vi "Log.vi"(7 "Message":string, 8 "error in (no error)":errorcluster, 10 "Level":T1, 11 "Logger in":refnum<class "Logger.lvclass">) -> (0 "error out":errorcluster, 3 "Logger out":refnum<class "Logger.lvclass">)   [LabVIEW 2022 SP3, in "Logger.lvlib" / "Logger.lvclass"]
uses:
  Logger.lvclass
  Logger.lvclass/Logger.ctl
  _Level.ctl
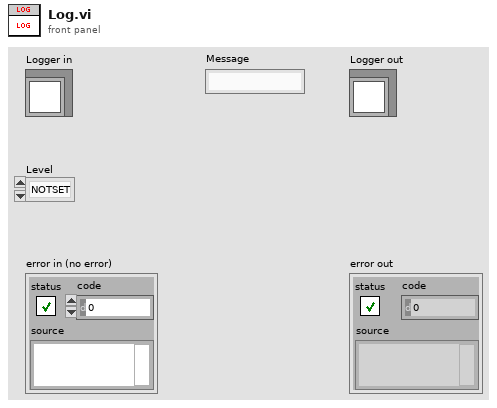
[diagram p1: front panel]
types:
  T1 = typedef "Logger.lvlib/Logger.lvclass/_Level.ctl" = enum16{"NOTSET", "DEBUG", "INFO", "WARNING", "ERROR", "CRITICAL"}
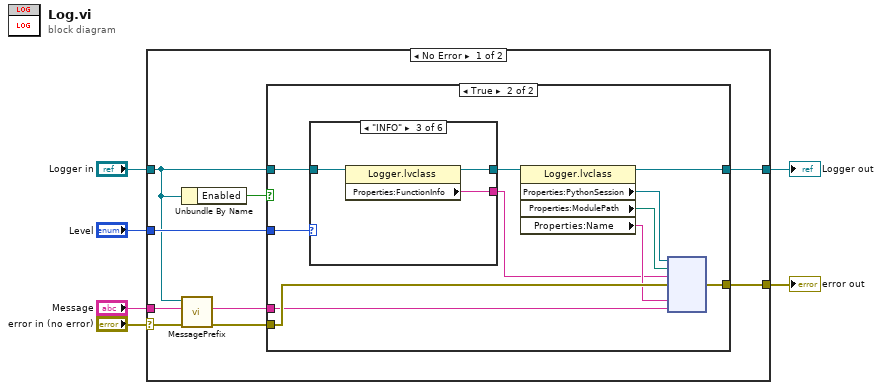
[diagram p0: block diagram]
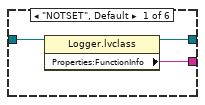
[diagram p3: hidden frame]
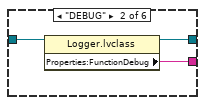
[diagram p4: hidden frame]
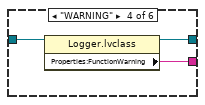
[diagram p5: hidden frame]
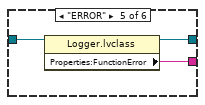
[diagram p6: hidden frame]
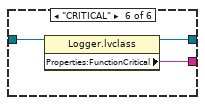
[diagram p7: hidden frame]
diagram:
  n1 = case shown="No Error" "error in (no error)" {
    selector: "error in (no error)" -> [w11 w48]
    tunnel: [w14 w48] -> w2
    tunnel: [w15 w47] -> w4
    tunnel: "Logger in" -> [w10 w47]
    tunnel: "Message" -> [w8 _]
    tunnel: "Level" -> [w12 _]
    frame No Error {
      n2 = Unbundle By Name(w10) -> ("Enabled"=w13:bool)
      n3 = call-dynamic "MessagePrefix.vi"("error in (no error)"=w11, "Message in"=w8, "Logger in"=w10) -> ("error out"=w7:errorcluster, "Message out"=w9:string)  [unwired: 6 in, 1 out]
      n4 = case shown="True" w13 {
        tunnel: [w17 w28] -> w15
        tunnel: w7 -> [w16 w27]
        tunnel: [w16 w26] -> w14
        tunnel: w9 -> [_ w23]
        tunnel: w10 -> [w17 w19]
        tunnel: w12 -> [_ w21]
        frame False {
        }
        frame True {
          n5 = case shown="\"INFO\"" w21 {
            tunnel: [w30 w33 w36 w39 w42 w45] -> w20
            tunnel: w19 -> [w31 w34 w37 w40 w43 w46]
            tunnel: [w29 w32 w35 w38 w41 w44] -> w18
            frame "NOTSET", Default {
              n6 = property class="Logger.lvclass"(reference=w31) -> (reference out=w30:refnum<class "Logger.lvclass">, "Properties:FunctionInfo"=w29:string)  [unwired: 1 in, 1 out]
            }
            frame "DEBUG" {
              n7 = property class="Logger.lvclass"(reference=w34) -> (reference out=w33:refnum<class "Logger.lvclass">, "Properties:FunctionDebug"=w32:string)  [unwired: 1 in, 1 out]
            }
            frame "INFO" {
              n8 = property class="Logger.lvclass"(reference=w37) -> (reference out=w36:refnum<class "Logger.lvclass">, "Properties:FunctionInfo"=w35:string)  [unwired: 1 in, 1 out]
            }
            frame "WARNING" {
              n9 = property class="Logger.lvclass"(reference=w40) -> (reference out=w39:refnum<class "Logger.lvclass">, "Properties:FunctionWarning"=w38:string)  [unwired: 1 in, 1 out]
            }
            frame "ERROR" {
              n10 = property class="Logger.lvclass"(reference=w43) -> (reference out=w42:refnum<class "Logger.lvclass">, "Properties:FunctionError"=w41:string)  [unwired: 1 in, 1 out]
            }
            frame "CRITICAL" {
              n11 = property class="Logger.lvclass"(reference=w46) -> (reference out=w45:refnum<class "Logger.lvclass">, "Properties:FunctionCritical"=w44:string)  [unwired: 1 in, 1 out]
            }
          }
          n12 = property class="Logger.lvclass"(reference=w20) -> (reference out=w28:refnum<class "Logger.lvclass">, "Properties:PythonSession"=w25:refnum<k35>, "Properties:ModulePath"=w24:path, "Properties:Name"=w22:string)  [unwired: 1 in, 1 out]
          n13 = node(w25, w24, w18, w27, w22, w23) -> (w26:errorcluster)  [unwired: 4 in, 3 out]
        }
      }
    }
    frame Error {
    }
  }
  "error out" <- w2
  "Logger out" <- w4
